vi "Convert Linear Ratio to dB.vi"(4 "X":dbl format="%.2f") -> (1 "dB":dbl format="%.2f")   [LabVIEW 2011]
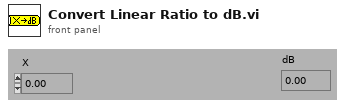
[diagram p1: front panel]
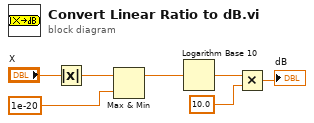
[diagram p0: block diagram]
diagram:
  n1 = Absolute Value(x="X") -> (abs(x)=w3:dbl)
  n2 = Max & Min(x=w3, y=1e-20) -> (max(x,y)=w1:dbl)  [unwired: 1 out]
  n3 = Logarithm Base 10(1:w1) -> (0:w7:dbl)
  n4 = Multiply(x=w7, y=10.0) -> (x*y=→"dB":dbl)
